vi "Division9225-7_FPGA.vi"(1 "y <+/-49,13>":fxp<+/-,49,13>, 2 "x <+/-40,4>":fxp<+/-,40,4>) -> (0 "x/y <+/-38,4>":fxp<+/-,48,14>)   [LabVIEW 2021]
uses:
  <vilib>/rvi/FXPMathLib/FxpDiv/subVIs/nifxpmath_Div_SimConfig.ctl
  <vilib>/rvi/FXPMathLib/FxpDiv/simVIs/DllFxpDivTemp_sub.vi
  <vilib>/rvi/FXPMathLib/FxpDiv/XNode/nifxpmath_Div.xnode
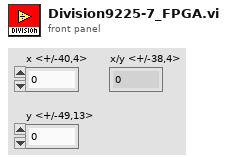
[diagram p1: front panel]
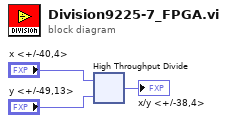
[diagram p0: block diagram]
diagram:
  n1 = xnode "High Throughput Divide"("x"="x <+/-40,4>", "y"="y <+/-49,13>") -> ("x/y"=→"x/y <+/-38,4>":fxp<+/-,48,14>)
